vi "Async Tx.vi"(8 "error in (no error)":errorcluster, 9 "framework iteration":u64, 10 "Dispatcher Interface in":refnum<class "Dispatcher Interface.lvclass">, 11 "Plugin Timing Group in":refnum<class "Plugin Timing.lvclass">) -> (0 "error out":errorcluster, 2 "Dispatcher Interface out":refnum<class "Dispatcher Interface.lvclass">, 3 "Plugin Timing Group out":refnum<class "Plugin Timing.lvclass">)   [LabVIEW 2017, in "DSF Core.lvlib" / "Scheduler Plugin Bundle.lvclass"]
uses:
  Scheduler/Scheduler Plugin Bundle.lvclass
  Timing.lvclass
  Interfaces/Dispatcher/Dispatcher Interface.lvclass
  Plugin Timing.lvclass
  C:/Git/DSF/Data Sharing Framework/Source/Core/Engine/Classes/Timing/Timing.lvclass
  Scheduler/Scheduler Transfer Group Bundle.lvclass
  Transfer Group Timing.lvclass
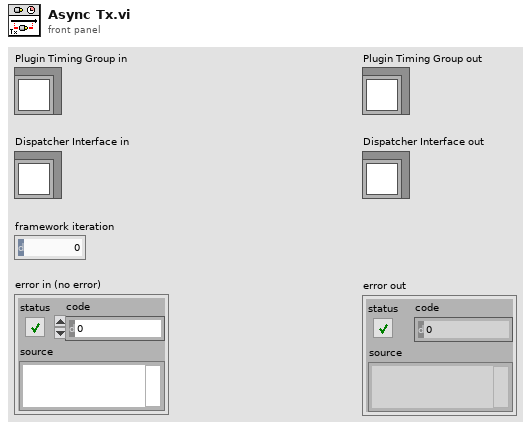
[diagram p1: front panel]
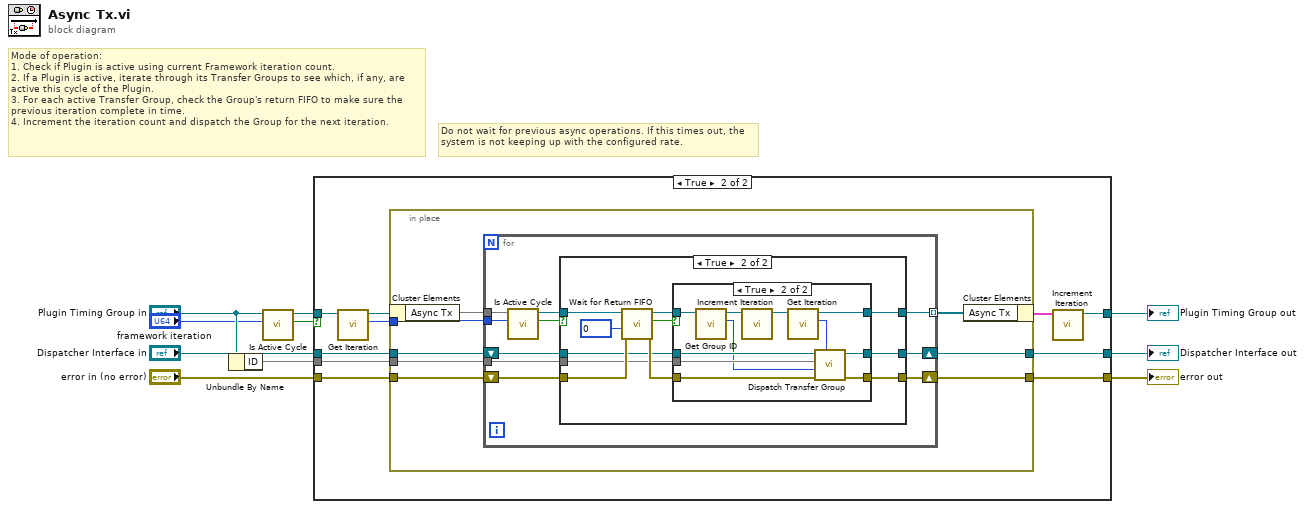
[diagram p0: block diagram]
diagram:
  # "Mode of operation:\n1. Check if Plugin is active using current Framework iteration count.\n2. If a Plugin is active, iterate through its Transfer Groups to see which, if any, are active this cycle of the Plugin.\n3. For each active Transfer Group, check the Group's return FIFO to make sure the previous iteration complete in time.\n4. Increment the iteration count and dispatch the Group for the next iteration."
  # "Do not wait for previous async operations. If this times out, the system is not keeping up with the configured rate."
  n1 = Unbundle By Name("Plugin Timing Group in") -> ("ID"=w5)
  n2 = call "Is Active Cycle.vi"("iteration"="framework iteration", "Timing in"="Plugin Timing Group in") -> ("active?"=w2:bool, "Timing out"=w3:refnum<class "Plugin Timing.lvclass">)  [unwired: 8 in]
  n3 = case shown="True" w2 {
    tunnel: [w13 w14] -> w10
    tunnel: "Dispatcher Interface in" -> [w12 w23]
    tunnel: [w12 w22] -> w8
    tunnel: "error in (no error)" -> [w11 w21]
    tunnel: [w11 w20] -> w6
    tunnel: w5 -> [_ w19]
    tunnel: w3 -> [w13 w18]
    frame False {
    }
    frame True {
      n4 = call "Get Iteration.vi"("Timing in"=w18) -> ("Iteration"=w16:u64, "Timing out"=w17:refnum<class "Plugin Timing.lvclass">)  [unwired: 9 in]
      n5 = in-place {
        in-place-border: w23 -> [w29]
        in-place-border: [w28] -> w22
        in-place-border: [w27] -> w20
        in-place-border: w21 -> [w26]
        in-place-border: w19 -> [w25]
        in-place-border: w16 -> [w24]
        n6 = in-place-cluster #1(w17) -> ("Async Tx"=w31)
        n7 = for {
          tunnel: w31 -> [w36]
          tunnel: [w32] -> w30 mode=indexing
          shift-right: [w40] -> w28
          shift-left: w29 -> [w41]
          shift-right: [w39] -> w27
          shift-left: w26 -> [w38]
          tunnel: w25 -> [w37]
          tunnel: w24 -> [w34]
          n8 = call "Is Active Cycle.vi"("iteration"=w34, "Timing in"=w36) -> ("active?"=w35:bool, "Timing out"=w33:refnum<class "Timing.lvclass">)  [unwired: 8 in]
          n9 = case shown="True" w35 {
            tunnel: w41 -> [w44 w48]
            tunnel: [w44 w53] -> w40
            tunnel: [w43 w52] -> w39
            tunnel: w38 -> [w43 w54]
            tunnel: w37 -> [_ w51]
            tunnel: w33 -> [w42 w50]
            tunnel: [w42 w45] -> w32
            frame False {
            }
            frame True {
              n10 = call "Wait for Return FIFO.vi"("error in (no error)"=w54, "timeout (0 ms)"=0, "Transfer Group Bundle in"=w50) -> ("error out"=w55:errorcluster, "iteration valid"=w46:bool, "Transfer Group Bundle out"=w47:refnum<class "Scheduler Transfer Group Bundle.lvclass">)  [unwired: 6 in]
              n11 = case shown="True" w46 {
                tunnel: [w57 w69] -> w53
                tunnel: [w56 w68] -> w52
                tunnel: w51 -> [_ w67]
                tunnel: w55 -> [w56 w66]
                tunnel: w48 -> [w57 w65]
                tunnel: w47 -> [w58 w61]
                tunnel: [w58 w62] -> w45
                frame False {
                }
                frame True {
                  n12 = call "Get Group ID.vi"("Transfer Group Timing in"=w61) -> ("Group ID"=w59:i32, "Transfer Group Timing out"=w60:refnum<class "Transfer Group Timing.lvclass">)  [unwired: 9 in]
                  n13 = call "Increment Iteration.vi"("Timing in"=w60) -> ("Timing out"=w64:refnum<class "Transfer Group Timing.lvclass">)  [unwired: 10 in]
                  n14 = call "Get Iteration.vi"("Timing in"=w64) -> ("Iteration"=w63:u64, "Timing out"=w62:refnum<class "Transfer Group Timing.lvclass">)  [unwired: 9 in]
                  n15 = call "Dispatch Transfer Group.vi"("Iteration"=w63, "error in (no error)"=w66, "Transfer Group ID"=w59, "Plugin ID"=w67, "Dispatcher Interface in"=w65) -> ("error out"=w68:errorcluster, "Dispatcher Interface out"=w69:refnum<class "Dispatcher Interface.lvclass">)  [unwired: 5 in]
                }
              }
            }
          }
        }
        n16 = in-place-cluster #1("Async Tx"=w30) -> (w15:cluster{})
      }
      n17 = call "Increment Iteration.vi"("Timing in"=w15) -> ("Timing out"=w14:refnum<class "Timing.lvclass">)  [unwired: 10 in]
    }
  }
  "Plugin Timing Group out" <- w10
  "Dispatcher Interface out" <- w8
  "error out" <- w6
